vi "replaceBallWhenGoOut.vi"(7 "Side":enum16{"Esquerdo", "Direito"}(ring) caption="Enum", 8 "error in (no error)":errorcluster, 9 "Game":refnum<class "Game.lvclass">, 10 "grSIM replacement":T1, 11 "Communication in":refnum<class "Communication.lvclass">) -> (0 "error out":errorcluster, 2 "grSIM replacement out":T1, 3 "Communication out":refnum<class "Communication.lvclass">, 5 "replaceBall":bool)   [LabVIEW 2023, in "Communication.lvclass"]
uses:
  Communication.lvclass
  Controls/grSimReplacement.ctl
  Paths/grSim Packet Command UDP Test Folder/grSim/grSim RobotReplacement.ctl
  Paths/grSim Packet Command UDP Test Folder/grSim/grSim_BallReplacement.ctl
  Game_class/Game.lvclass
  Game_class/Game.lvclass/Game.ctl
  Events_class/Events.lvclass/Events.ctl
  Object_class/Object.lvclass/Object.ctl
  Object_class/Read x.vi
  Object_class/Read position(x,y).vi
  Object_class/Read y.vi
  Game_class/Read FieldRef.vi
  Game_class/Read BallRef.vi
  Game_class/Read EventsRef.vi
  Events_class/Read ball_out.vi
  Ball_class/Ball.lvclass
  C:/Users/lucio/Desktop/roboime/SSL_AI/Object_class/Object.lvclass
  Field_class/Field.lvclass
  Events_class/Events.lvclass
  Utilities_class/Utilities.lvclass
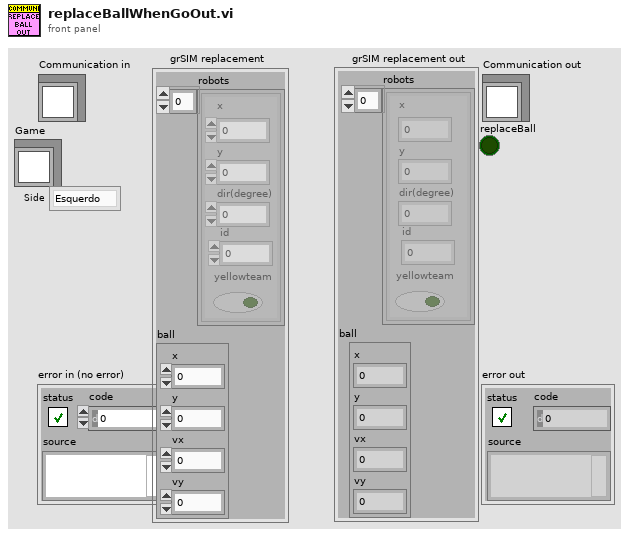
[diagram p1: front panel]
types:
  T1 = typedef "grSimReplacement.ctl" = cluster{"robots":T2[], "ball":T3}
  T2 = typedef "grSim RobotReplacement.ctl" = cluster{"x":dbl, "y":dbl, "dir(degree)":dbl, "yellowteam":bool, "id":u32}
  T3 = typedef "grSim_BallReplacement.ctl" = cluster{"x":dbl, "y":dbl, "vx":dbl, "vy":dbl}
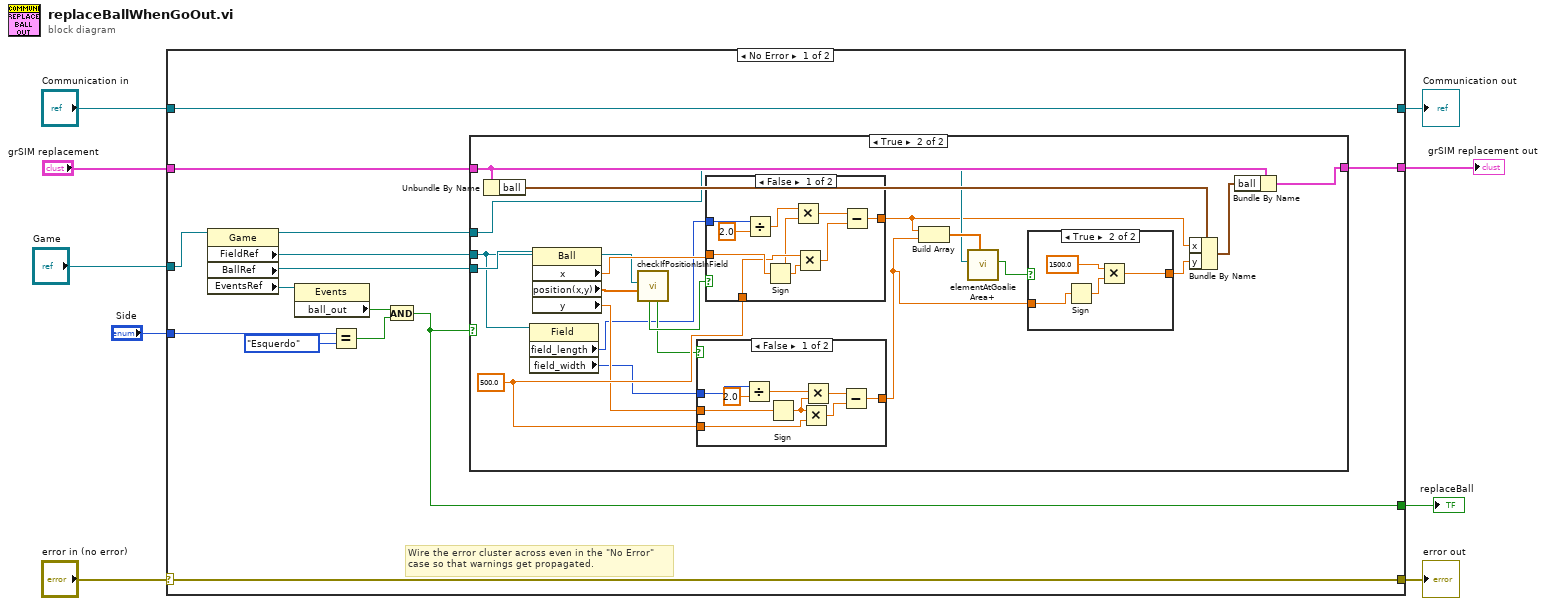
[diagram p0: block diagram]
diagram:
  n1 = case shown="No Error" "error in (no error)" {
    selector: "error in (no error)" -> [w22 w71]
    tunnel: [w22 w71] -> w8
    tunnel: [w23 w70] -> w6
    tunnel: "Communication in" -> [w23 w70]
    tunnel: "Game" -> [w21 _]
    tunnel: "grSIM replacement" -> [w19 _]
    tunnel: [w18 _] -> w3
    tunnel: [w14 _] -> w2
    tunnel: "Side" -> [w12 _]
    frame No Error {
      # "Wire the error cluster across even in the \"No Error\"\ncase so that warnings get propagated."
      n2 = property class="Game"(reference=w21) -> (reference out=w10:refnum<class "Game.lvclass">, "FieldRef"=w16:refnum<class "Field.lvclass">, "BallRef"=w17:refnum<class "Ball.lvclass">, "EventsRef"=w20:refnum<class "Events.lvclass">)  [unwired: 1 in, 1 out]
      n3 = property class="Events"(reference=w20) -> ("ball_out"=w15:bool)  [unwired: 1 in, 2 out]
      n4 = Equal?(x=w12, y=enum16{"Esquerdo", "Direito"}."Esquerdo") -> (x = y?=w13:bool)
      n5 = And(x=w15, y=w13) -> (x .and. y?=w14:bool)
      n6 = case shown="True" w14 {
        tunnel: [w24 w44] -> w18
        tunnel: w19 -> [w24 w43]
        tunnel: w17 -> [_ w40]
        tunnel: w16 -> [_ w36]
        tunnel: w10 -> [_ w29]
        frame False {
        }
        frame True {
          w35 = 500.0 ("x")
          n7 = Unbundle By Name(w43) -> ("ball"=w42:T3)
          n8 = property class="Field"(reference=w36) -> ("field_length"=w31:i32, "field_width"=w32:i32)  [unwired: 1 in, 2 out]
          n9 = property class="Ball"(reference=w40) -> ("x"=w38:dbl, "position(x,y)"=w39:dbl[], "y"=w34:dbl)  [unwired: 1 in, 2 out]
          n10 = call "checkIfPositionIsInField.vi"("Position"=w39, "FieldRef"=w36) -> ("y Is in Field?"=w33:bool, "x Is in Field?"=w37:bool)  [unwired: 5 in, 3 out]
          n11 = case shown="False" w33 {
            tunnel: w35 -> [w57 _]
            tunnel: w34 -> [w55 w59]
            tunnel: [w56 w59] -> w25
            tunnel: w32 -> [w54 _]
            frame False {
              n12 = Divide(x=w54, y=2.0 ("x")) -> (x/y=w52:dbl)
              n13 = Sign(1:w55) -> (0:w50:dbl)
              n14 = Multiply(x=w50, y=w57) -> (x*y=w58:dbl)
              n15 = Multiply(x=w52, y=w50) -> (x*y=w51:dbl)
              n16 = Subtract(x=w51, y=w58) -> (x-y=w56:dbl)
            }
            frame True {
            }
          }
          n17 = case shown="False" w37 {
            tunnel: [w66 w69] -> w28
            tunnel: w38 -> [w68 w69]
            tunnel: w35 -> [w67 _]
            tunnel: w31 -> [w64 _]
            frame False {
              n18 = Divide(x=w64, y=2.0 ("x")) -> (x/y=w62:dbl)
              n19 = Sign(1:w68) -> (0:w61:dbl)
              n20 = Multiply(x=w62, y=w61) -> (x*y=w60:dbl)
              n21 = Multiply(x=w67, y=w61) -> (x*y=w65:dbl)
              n22 = Subtract(x=w60, y=w65) -> (x-y=w66:dbl)
            }
            frame True {
            }
          }
          n23 = Build Array(w28, w25) -> (w30:dbl[])
          n24 = call "elementAtGoalieArea+.vi"("Elemento pos."=w30, "Game"=w29) -> ("Elemento at goalkeeper area + ?"=w27:bool)  [unwired: 7 in, 2 out]
          n25 = case shown="True" w27 {
            tunnel: [w45 w46] -> w26
            tunnel: w25 -> [w45 w48]
            frame False {
            }
            frame True {
              n26 = Sign(1:w48) -> (0:w47:dbl)
              n27 = Multiply(x=1500.0, y=w47) -> (x*y=w46:dbl)
            }
          }
          n28 = Bundle By Name(cluster=w42, "x"=w28, "y"=w26) -> (w41:T3)
          n29 = Bundle By Name(cluster=w43, "ball"=w41) -> (w44:T1)
        }
      }
    }
    frame Error {
    }
  }
  "error out" <- w8
  "Communication out" <- w6
  "grSIM replacement out" <- w3
  "replaceBall" <- w2
